vi "Read Config.vi"(8 "error in (no error)":errorcluster) -> (0 "error out":errorcluster, 3 "Config":T1)   [LabVIEW 2020]
uses:
  ctl/Config Cluster.ctl
  <vilib>/Utility/config.llb/Read Key (String).vi
  <vilib>/Utility/config.llb/Read Key (Double).vi
  <vilib>/Utility/config.llb/Read Key (Boolean).vi
  <vilib>/Utility/config.llb/Read Key (Path).vi
  <vilib>/Utility/config.llb/NI_LVConfig.lvlib
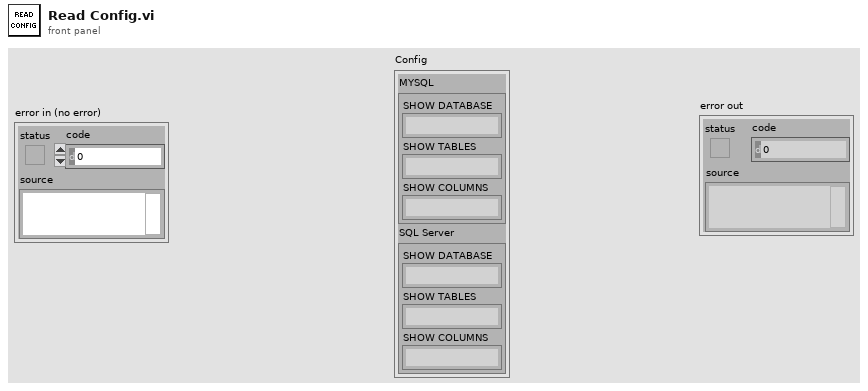
[diagram p1: front panel]
types:
  T1 = typedef "Config Cluster.ctl" = cluster{"MYSQL":cluster{"SHOW DATABASE":string, "SHOW TABLES":string, "SHOW COLUMNS":string}, "SQL Server":cluster{"SHOW DATABASE":string, "SHOW TABLES":string, "SHOW COLUMNS":string}}
  T2 = typedef "NI_LVConfig.lvlib/Config Data RefNum.ctl" = refnum<k1>
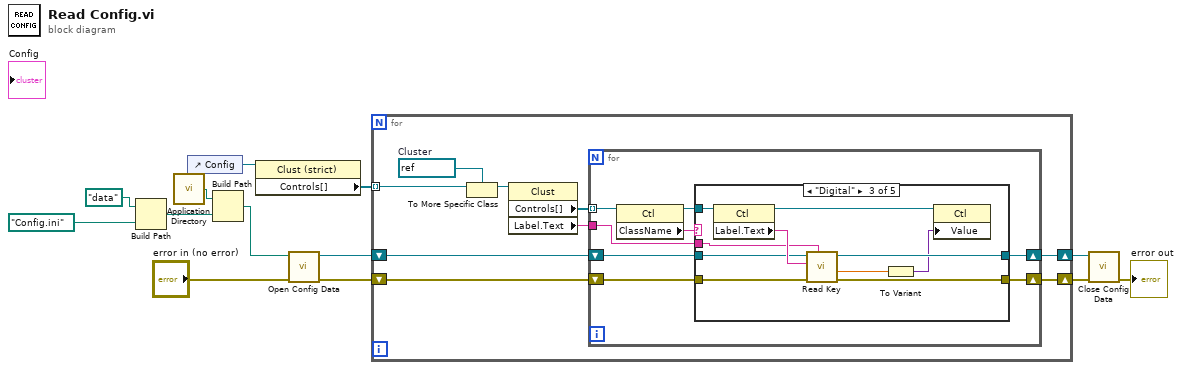
[diagram p0: block diagram]
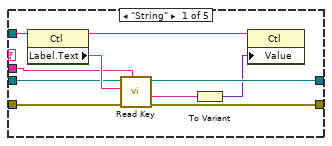
[diagram p2: hidden frame]
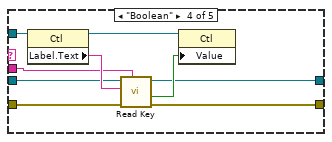
[diagram p4: hidden frame]
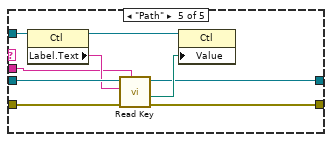
[diagram p5: hidden frame]
diagram:
  n1 = Build Path(base path=path "data", name or relative path=path "Config.ini") -> (appended path=w7:path)
  n2 = call <vilib>:"Application Directory.vi"() -> ("Application Directory"=w13:path)
  n3 = control-ref of="Config"() -> (w3:refnum<vi>)
  n4 = Build Path(base path=w13, name or relative path=w7) -> (appended path=w12:path)
  n5 = property class="Clust (strict)"(reference=w3) -> ("Controls[]"=w2:refnum<vi>[])  [unwired: 1 in, 2 out]
  n6 = call <vilib>:"Open Config Data.vi"("error in (no error)"="error in (no error)", "configuration file path"=w12) -> ("error out"=w8:errorcluster, "refnum"=w9:T2)  [unwired: 7 in, 1 out]
  n7 = for {
    tunnel: w2 -> [w14] mode=indexing
    shift-right: [w21] -> w10
    shift-left: w9 -> [w20]
    shift-right: [w22] -> w11
    shift-left: w8 -> [w19]
    w18 = refnum<vi> refnum  # Cluster
    n8 = To More Specific Class(target class=w18, reference=w14) -> (specific class reference=w17:refnum<vi>)  [unwired: 1 in, 1 out]
    n9 = property class="Clust"(reference=w17) -> ("Controls[]"=w16:refnum<vi>[], "Label.Text"=w15:string)  [unwired: 1 in, 2 out]
    n10 = for {
      tunnel: w16 -> [w24] mode=indexing
      tunnel: w15 -> [w23]
      shift-right: [w26] -> w21
      shift-left: w20 -> [w29]
      shift-right: [w25] -> w22
      shift-left: w19 -> [w28]
      n11 = property class="Ctl"(reference=w24) -> (reference out=w27:refnum<vi>, "ClassName"=w30:string)  [unwired: 1 in, 1 out]
      n12 = case shown="\"Digital\"" w30 {
        tunnel: w29 -> [w36 w42 w49 w57 w69]
        tunnel: w28 -> [w37 w41 w48 w56 w68]
        tunnel: w27 -> [w38 _ w50 w58 w70]
        tunnel: [w35 w42 w47 w55 w64] -> w26
        tunnel: [w34 w41 w46 w54 w63] -> w25
        tunnel: w23 -> [w31 _ w45 w53 w62]
        frame "String" {
          n13 = property class="Ctl"(reference=w38) -> (reference out=w39:refnum<vi>, "Label.Text"=w40:string)  [unwired: 1 in, 1 out]
          n14 = call-poly <vilib>:"Read Key.vi"("section"=w31, "error in (no error)"=w37, "key"=w40, "refnum"=w36) -> ("error out"=w34:errorcluster, "value"=w32:string, "refnum out"=w35:T2)  [unwired: 4 in, 1 out]
          n15 = To Variant(anything=w32) -> (Variant=w33:variant)
          n16 = property class="Ctl"(reference=w39, "Value"=w33) -> ()  [unwired: 1 in, 2 out]
        }
        frame "", Default {
        }
        frame "Digital" {
          n17 = property class="Ctl"(reference=w50) -> (reference out=w51:refnum<vi>, "Label.Text"=w52:string)  [unwired: 1 in, 1 out]
          n18 = call-poly <vilib>:"Read Key.vi"("section"=w45, "error in (no error)"=w48, "key"=w52, "refnum"=w49) -> ("error out"=w46:errorcluster, "value"=w43:dbl, "refnum out"=w47:T2)  [unwired: 4 in, 1 out]
          n19 = To Variant(anything=w43) -> (Variant=w44:variant)
          n20 = property class="Ctl"(reference=w51, "Value"=w44) -> ()  [unwired: 1 in, 2 out]
        }
        frame "Boolean" {
          n21 = property class="Ctl"(reference=w58) -> (reference out=w60:refnum<vi>, "Label.Text"=w61:string)  [unwired: 1 in, 1 out]
          n22 = call-poly <vilib>:"Read Key.vi"("section"=w53, "error in (no error)"=w56, "key"=w61, "refnum"=w57) -> ("error out"=w54:errorcluster, "value"=w59:bool, "refnum out"=w55:T2)  [unwired: 4 in, 1 out]
          n23 = property class="Ctl"(reference=w60, "Value"=w59) -> ()  [unwired: 1 in, 2 out]
        }
        frame "Path" {
          n24 = property class="Ctl"(reference=w70) -> (reference out=w66:refnum<vi>, "Label.Text"=w67:string)  [unwired: 1 in, 1 out]
          n25 = call-poly <vilib>:"Read Key.vi"("section"=w62, "error in (no error)"=w68, "key"=w67, "refnum"=w69) -> ("error out"=w63:errorcluster, "value"=w65:path, "refnum out"=w64:T2)  [unwired: 4 in, 1 out]
          n26 = property class="Ctl"(reference=w66, "Value"=w65) -> ()  [unwired: 1 in, 2 out]
        }
      }
    }
  }
  n27 = call <vilib>:"Close Config Data.vi"("error in (no error)"=w11, "refnum"=w10) -> ("error out"=→"error out":errorcluster)  [unwired: 8 in, 1 out]
